vi "Auto VideoMode.vi"(1 "Resolution":T1=1 items=["Low", "Med.", "High", "Max."], 2 "Camera":T2="Travcam") -> (0 "VideoMode":u32)   [LabVIEW 2015]
uses:
  Camera enum/Camera enum.ctl
  Camera enum/Camera resolution.ctl
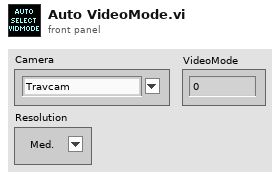
[diagram p1: front panel]
types:
  T1 = typedef "Camera resolution.ctl" = u8
  T2 = typedef "Camera enum.ctl" = string
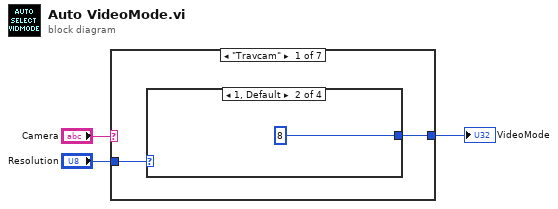
[diagram p0: block diagram]
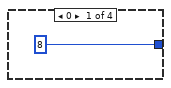
[diagram p2: hidden frame]
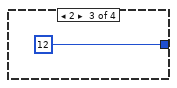
[diagram p3: hidden frame]
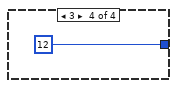
[diagram p4: hidden frame]
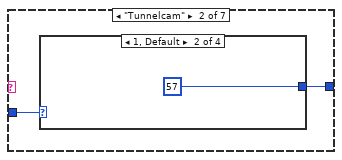
[diagram p5: hidden frame]
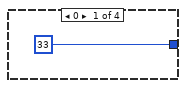
[diagram p6: hidden frame]
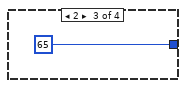
[diagram p7: hidden frame]
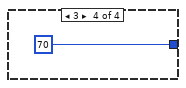
[diagram p8: hidden frame]
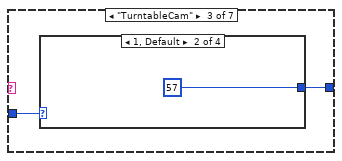
[diagram p9: hidden frame]
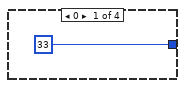
[diagram p10: hidden frame]
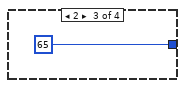
[diagram p11: hidden frame]
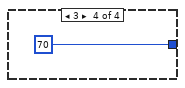
[diagram p12: hidden frame]
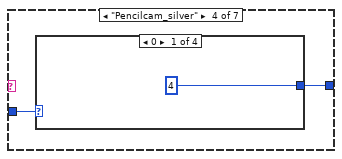
[diagram p13: hidden frame]
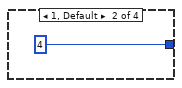
[diagram p14: hidden frame]
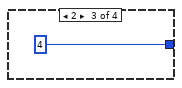
[diagram p15: hidden frame]
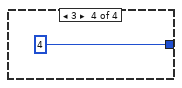
[diagram p16: hidden frame]
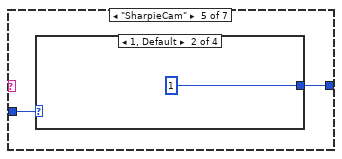
[diagram p17: hidden frame]
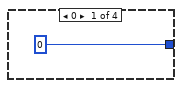
[diagram p18: hidden frame]
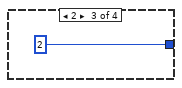
[diagram p19: hidden frame]
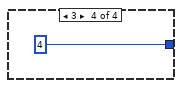
[diagram p20: hidden frame]
diagram:
  n1 = case shown="\"Travcam\"" "Camera" {
    tunnel: [w5 w11 w17 w23 w29 w35 u32 0] -> w3
    tunnel: "Resolution" -> [w4 w10 w16 w22 w28 w34 _]
    frame "Travcam" {
      n2 = case shown="1, Default" w4 {
        tunnel: [u32 8 u32 8 u32 12 u32 12] -> w5
        frame 0 {
        }
        frame 1, Default {
        }
        frame 2 {
        }
        frame 3 {
        }
      }
    }
    frame "Tunnelcam" {
      n3 = case shown="1, Default" w10 {
        tunnel: [u32 33 u32 57 u32 65 u32 70] -> w11
        frame 0 {
        }
        frame 1, Default {
        }
        frame 2 {
        }
        frame 3 {
        }
      }
    }
    frame "TurntableCam" {
      n4 = case shown="1, Default" w16 {
        tunnel: [u32 33 u32 57 u32 65 u32 70] -> w17
        frame 0 {
        }
        frame 1, Default {
        }
        frame 2 {
        }
        frame 3 {
        }
      }
    }
    frame "Pencilcam_silver" {
      n5 = case shown="0" w22 {
        tunnel: [u32 4 u32 4 u32 4 u32 4] -> w23
        frame 0 {
        }
        frame 1, Default {
        }
        frame 2 {
        }
        frame 3 {
        }
      }
    }
    frame "SharpieCam" {
      n6 = case shown="1, Default" w28 {
        tunnel: [u32 0 u32 1 u32 2 u32 4] -> w29
        frame 0 {
        }
        frame 1, Default {
        }
        frame 2 {
        }
        frame 3 {
        }
      }
    }
    frame "Microscope" {
      n7 = case shown="1, Default" w34 {
        tunnel: [u32 2 u32 2 u32 4 u32 4] -> w35
        frame 0 {
        }
        frame 1, Default {
        }
        frame 2 {
        }
        frame 3 {
        }
      }
    }
    frame Default {
    }
  }
  "VideoMode" <- w3
